vi "RT Loop - VIDEO.vi"(8 "error in (no error)":errorcluster, 9 "trigger":bool, 10 "Video RT FIFO in":refnum<k33>, 11 "Message Queue":refnum<queue>) -> ()   [LabVIEW 2017]
doc: "Read and analyze acceleration waveform data from FPGA via DMA FIFO. If the acceleration is over the limit, then send the acceleration waveform data to the Log Data Loop."
uses:
  support/Message Queue/Message Cluster.ctl
  <vilib>/vision/Image Controls.llb/IMAQ Image.ctl
  <vilib>/userdefined/High Color/IMAQdx.ctl
  <vilib>/vision/Avi.llb/IMAQ AVI2 Codec Path.ctl
  Globals/Global - All RT Loop Stop.vi
  <vilib>/vision/driver/NI_Vision_Acquisition_Software.lvlib
  support/Message Queue/Message Queue.lvlib
panel:
  out "Video RT FIFO 2":refnum<k33>
  out "Webcam":T1(plugin-control)
  in  "stop":bool
  out "Codec Names":string[](array[string])
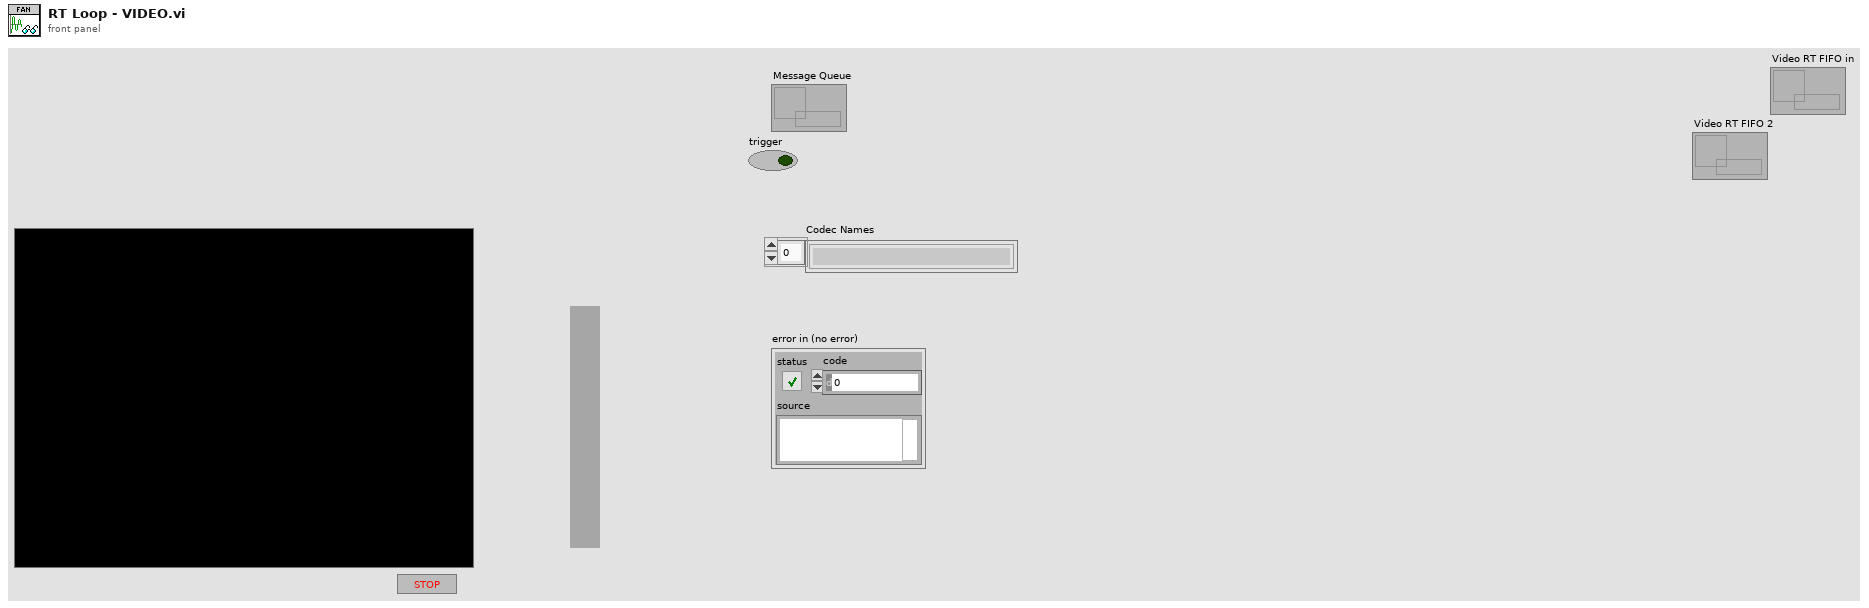
[diagram p1: front panel]
types:
  T1 = typedef "IMAQ Image.ctl" = refnum<image>
  T2 = typedef "IMAQdx.ctl" = refnum<k21>
  T3 = typedef "Image Type" = u32
  T4 = typedef "IMAQ AVI2 Codec Path.ctl" = u32
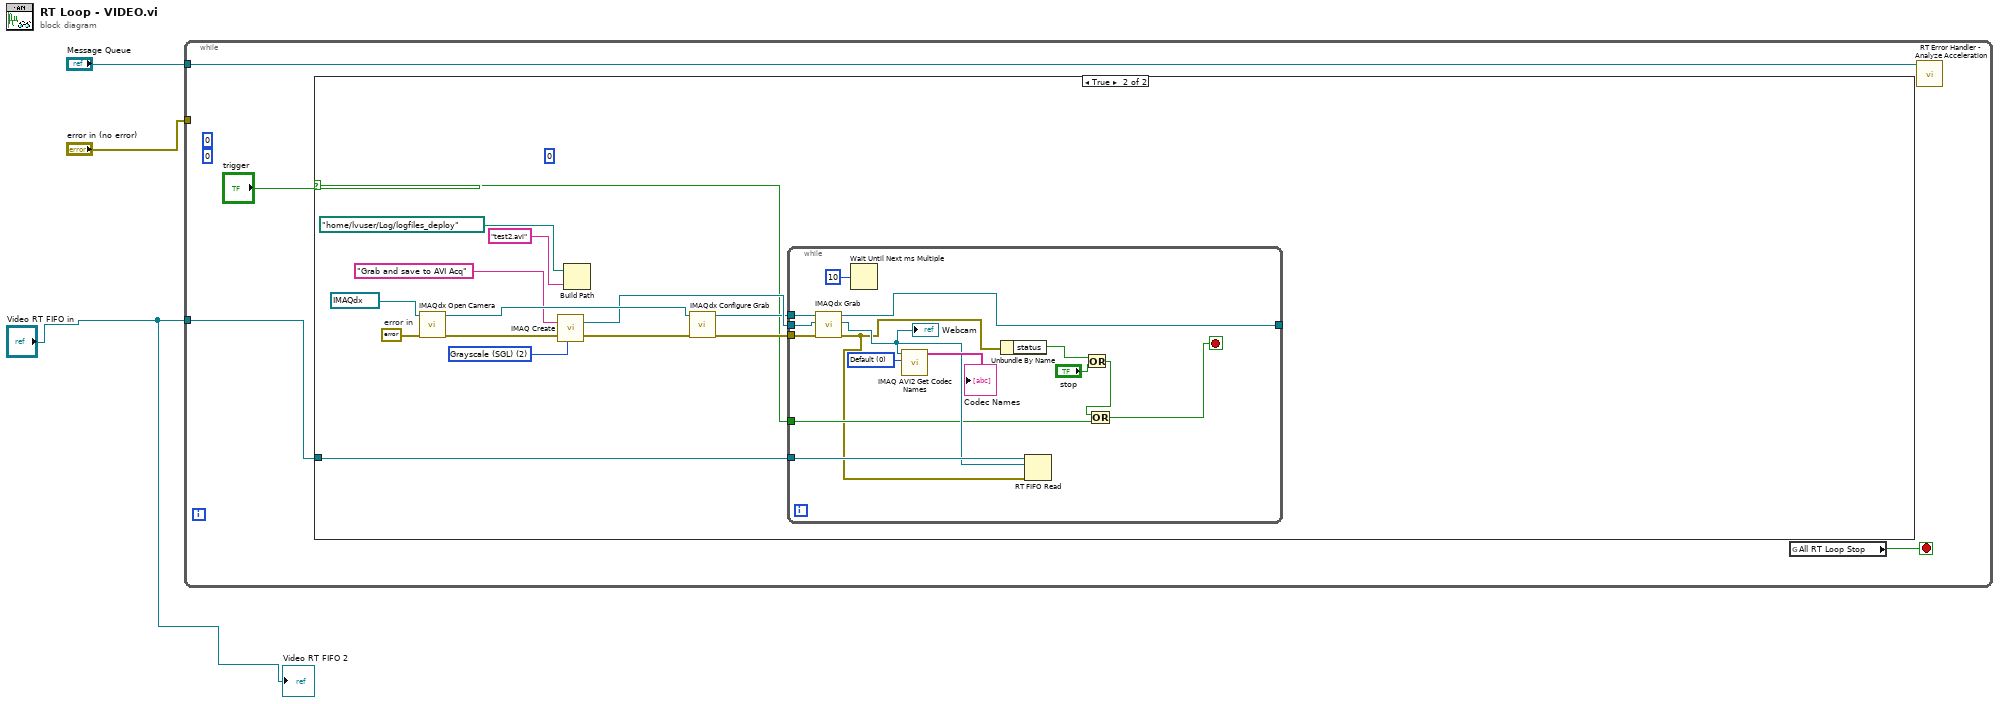
[diagram p0: block diagram]
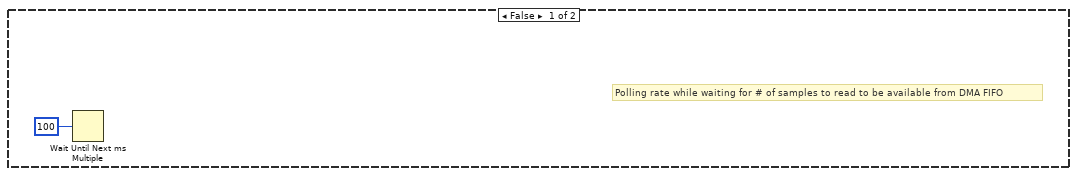
[diagram p2: hidden frame]
diagram:
  n1 = while {
    tunnel: "error in (no error)" -> [_]
    tunnel: "Message Queue" -> [w6]
    tunnel: "Video RT FIFO in" -> [w4]
    stop <- w7 stop-if-true
    (unwired) u32 0 ("Number of Elements")
    (unwired) 0 ("Timeout (ms)")
    n2 = case shown="True" "trigger" {
      selector: "trigger" -> [_ w9]
      tunnel: w4 -> [_ w11]
      frame False {
        # "Polling rate while waiting for # of samples to read to be available from DMA FIFO"
        n3 = Wait Until Next ms Multiple(millisecond multiple=u32 100) -> ()  [unwired: 1 out]
      }
      frame True {
        w14 = T3 2 items=["Grayscale (U8)", "Grayscale (I16)", "Grayscale (SGL)", "Complex (CSG)", "RGB (U32)", "HSL (U32)", "RGB (U64)", "Grayscale (U16)"] ("Image Type")
        w18 = errorcluster {"status"=FALSE, "code"=0, "source"=""}  # error in
        (unwired) 0 ("Timeout (ms)")
        n4 = call <vilib>:"IMAQdx Open Camera.vi"("error in"=w18, "Session In"=T2 "cam0") -> ("error out"=w13:errorcluster, "Session Out"=w22:T2)  [unwired: 8 in]
        n5 = call "IMAQ Create"("Image Name"="Grab and save to AVI Acq", "Image Type"=w14, "error in (no error)"=w13) -> ("New Image"=w19:T1, "error out"=w10:errorcluster)  [unwired: 2 in]
        n6 = Build Path(base path=path "/home/lvuser/Log/logfiles_deploy" ("AVI Path"), name or relative path="test2.avi") -> ()  [unwired: 1 out]
        n7 = call <vilib>:"IMAQdx Configure Grab.vi"("error in"=w10, "Session In"=w22) -> ("error out"=w20:errorcluster, "Session Out"=w12:T2)  [unwired: 8 in]
        n8 = while {
          tunnel: w20 -> [w37]
          tunnel: w12 -> [w36]
          tunnel: w19 -> [w35]
          tunnel: [w34] -> _
          tunnel: w11 -> [w29]
          tunnel: w9 -> [w26]
          stop <- w24 stop-if-true
          w31 = T4 0 items=["Default", "System", "Built in Vision"] ("Codec Source")
          n9 = call <vilib>:"IMAQdx Grab.vi"("error in"=w37, "Image In"=w35, "Session In"=w36) -> ("error out"=w23:errorcluster, "Image Out"=w28:T1, "Session Out"=w34:T2)  [unwired: 5 in, 1 out]
          "Webcam" <- w28
          n10 = Wait Until Next ms Multiple(millisecond multiple=u32 10 ("milliseconds to wait")) -> ()  [unwired: 1 out]
          n11 = call "IMAQ AVI2 Get Codec Names"("Codec Source"=w31, "Image"=w28) -> ("Codec Names"=→"Codec Names":string[])  [unwired: 8 in, 1 out]
          n12 = Unbundle By Name(w23) -> ("status"=w27:bool)
          n13 = RT FIFO Read(0:w29, 1:w28, 3:w23) -> ()  [unwired: 1 in, 5 out]
          n14 = Or(x=w27, y="stop") -> (x .or. y?=w25:bool)
          n15 = Or(x=w25, y=w26) -> (x .or. y?=w24:bool)
        }
      }
    }
    n16 = global read "Global - All RT Loop Stop.vi" "All RT Loop Stop"() -> (w7:bool)
    n17 = call "RT Error Handler - Analyze Acceleration.vi"("Message Queue"=w6) -> ()  [unwired: 10 in, 1 out]
  }
  "Video RT FIFO 2" <- "Video RT FIFO in"
